vi "DrawText.vi"(0 "reference in":refnum<class "LcPictureBox.lvclass">, 1 "Origin":cluster{"X":sgl, "Y":sgl}, 2 "Alignment(Left,Top)":T2, 3 "Text":string, 5 "Error In":errorcluster, 6 "Font(Arial,14pts,Regular)":T1={"FontName"="Arial", "Size(Pts)"=14.0, "Style"=enum."Regular"}, 7 "Color(Black)":u32(colorbox), 8 "SmoothingMode((AntiAlias))":T3=enum."AntiAlias", 9 "Alpha(100%)":dbl=100.0 min=0.0 max=100.0 format="%#_g%%", 10 "BgColor(Transparent)":u32(colorbox)=16777216) -> (14 "reference out":refnum<class "LcPictureBox.lvclass">, 19 "Error Out":errorcluster)   [LabVIEW 2020, in "LcPictureBox.lvclass"]
uses:
  <userlib>/_LabVIEWCommon/LcPictureBox_class/LcPictureBox.lvclass
  <userlib>/_LabVIEWCommon/LcPictureBox_class/SmoothingMode.ctl
  <userlib>/_LabVIEWCommon/LcPictureBox_class/Font.ctl
  System.Drawing
  <userlib>/_LabVIEWCommon/LcPictureBox_class/LcPictureBox.lvclass/LcPictureBox.ctl
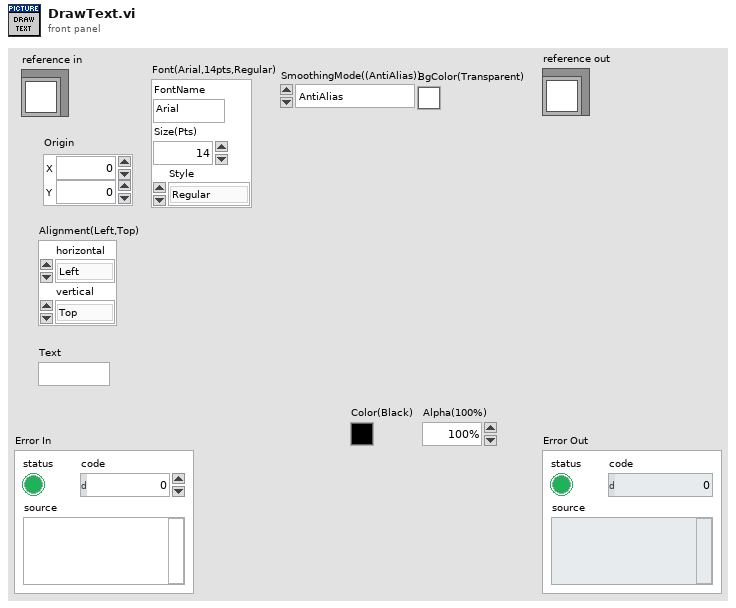
[diagram p1: front panel]
types:
  T1 = typedef "LcPictureBox.lvclass/Font.ctl" = cluster{"FontName":string, "Size(Pts)":dbl, "Style":enum16{"Regular", "Bold", "Italic", "Underline", "Strikeout"}}
  T2 = cluster{"horizontal":enum16{"Left", "Center", "Right"}, "vertical":enum16{"Top", "Center", "Bottom"}}
  T3 = typedef "LcPictureBox.lvclass/SmoothingMode.ctl" = enum16{"None", "HighSpeed", "HighQuality", "AntiAlias"}
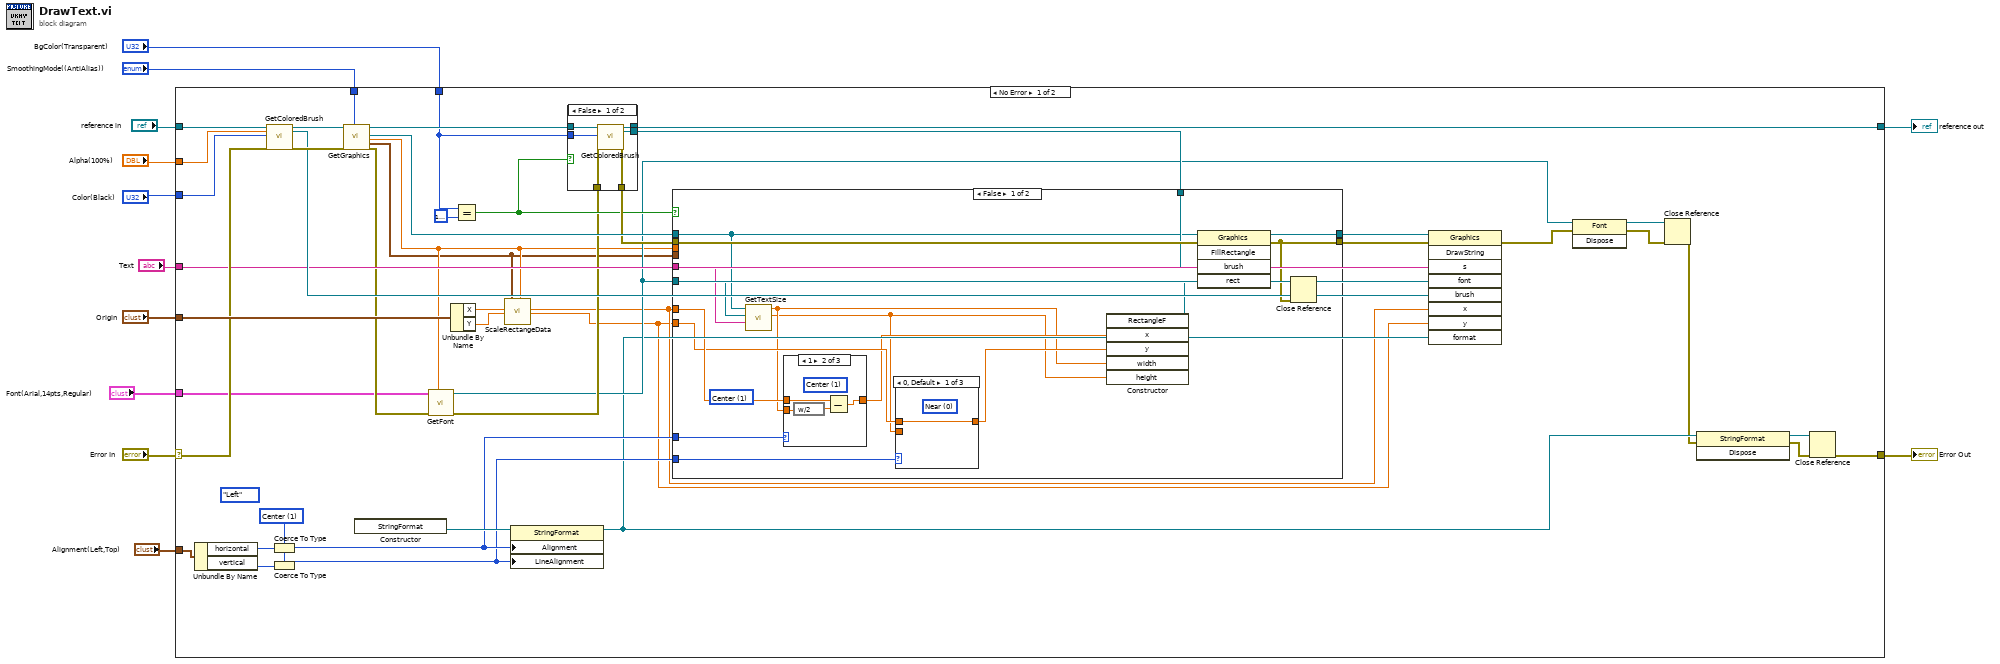
[diagram p0: block diagram]
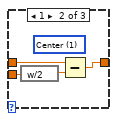
[diagram p2: hidden frame]
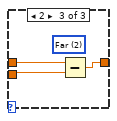
[diagram p3: hidden frame]
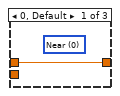
[diagram p4: hidden frame]
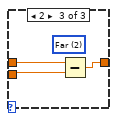
[diagram p5: hidden frame]
diagram:
  n1 = case shown="No Error" "Error In" {
    selector: "Error In" -> [w54 w101]
    tunnel: [w29 w101] -> w11
    tunnel: [w37 w100] -> w10
    tunnel: "reference in" -> [w56 w100]
    tunnel: "SmoothingMode((AntiAlias))" -> [w50 _]
    tunnel: "Color(Black)" -> [w52 _]
    tunnel: "Alpha(100%)" -> [w53 _]
    tunnel: "Origin" -> [w57 _]
    tunnel: "Text" -> [w48 _]
    tunnel: "Alignment(Left,Top)" -> [w45 _]
    tunnel: "Font(Arial,14pts,Regular)" -> [w41 _]
    tunnel: "BgColor(Transparent)" -> [w35 _]
    frame No Error {
      (unwired) enum16{"Left", "Center", "Right"}."Left" ("horizontal")
      w42 = 1 items=["Near", "Center", "Far"] ("Alignment")
      n2 = Unbundle By Name(w45) -> ("horizontal"=w44:enum16{"Left", "Center", "Right"}, "vertical"=w43:enum16{"Top", "Center", "Bottom"})
      n3 = call <userlib>:"GetColoredBrush.vi"("reference in"=w56, "Alpha(100%)"=w53, "Color(Black)"=w52, "Error In"=w54) -> ("reference out"=w55:refnum<class "LcPictureBox.lvclass">, "SolidBrushRef"=w49:refnum<k24>, "Error Out"=w51:errorcluster)  [unwired: 13 in]
      n4 = Coerce To Type(0:w44, 1:w42) -> (2:w31:i32)
      n5 = Coerce To Type(0:w43, 1:w42) -> (2:w30:i32)
      n6 = call <userlib>:"GetGraphics.vi"("LcPictureBox in"=w55, "error in (no error)"=w51, "SmoothingMode"=w50) -> ("LcPictureBox out"=w38:refnum<class "LcPictureBox.lvclass">, "Graphics"=w40:refnum<k24>, "Scale"=w16:dbl, "Offset"=w15:cluster{"x":sgl, "y":sgl}, "error out"=w47:errorcluster)  [unwired: 12 in]
      n7 = constructor class="StringFormat"() -> (reference out=w46:refnum<k24>)  [unwired: 3 in, 2 out]
      n8 = call <userlib>:"GetFont.vi"("Scale"=w16, "error in (no error)"=w47, "Font(Arial,14pts,Regular)"=w41) -> ("error out"=w32:errorcluster, "Font"=w28:refnum<k24>)  [unwired: 7 in]
      n9 = Unbundle By Name(w57) -> ("X"=w20:sgl, "Y"=w18:sgl)
      n10 = Equal?(x=w35, y=u32 16777216) -> (x = y?=w34:bool)
      n11 = call <userlib>:"ScaleRectangeData.vi"("X-In"=w20, "Y-In"=w18, "Offset(raw)"=w15, "Scale"=w16) -> ("X-Out"=w19:sgl, "Y-Out"=w17:sgl)  [unwired: 12 in, 2 out]
      n12 = property class="StringFormat"(reference=w46, "Alignment"=w31, "LineAlignment"=w30) -> (reference out=w24:refnum<k24>)  [unwired: 1 in, 1 out]
      n13 = case shown="False" w34 {
        tunnel: w38 -> [w97 w99]
        tunnel: [w96 w99] -> w37
        tunnel: w32 -> [w95 w98]
        tunnel: [w94 w98] -> w36
        tunnel: w35 -> [w93 _]
        tunnel: [w92 _] -> w33
        frame False {
          n14 = call <userlib>:"GetColoredBrush.vi"("reference in"=w97, "Color(Black)"=w93, "Error In"=w95) -> ("reference out"=w96:refnum<class "LcPictureBox.lvclass">, "SolidBrushRef"=w92:refnum<k24>, "Error Out"=w94:errorcluster)  [unwired: 14 in]
        }
        frame True {
        }
      }
      n15 = case shown="False" w34 {
        tunnel: w36 -> [w73 w90]
        tunnel: w40 -> [w68 w91]
        tunnel: [w72 w91] -> w14
        tunnel: [w63 w90] -> w13
        tunnel: w33 -> [w71 _]
        tunnel: w48 -> [w69 _]
        tunnel: w28 -> [w70 _]
        tunnel: w19 -> [w66 _]
        tunnel: w17 -> [w64 _]
        tunnel: w31 -> [w67 _]
        tunnel: w30 -> [w65 _]
        tunnel: w15 -> [_ _]
        tunnel: w16 -> [_ _]
        frame False {
          (unwired) 1 items=["Near", "Center", "Far"] ("Alignment")
          n16 = call <userlib>:"GetTextSize.vi"("Text"=w69, "Font"=w70, "Graphics"=w68) -> ("Height"=w58:sgl, "Width"=w59:sgl)  [unwired: 6 in, 1 out]
          n17 = case shown="1" w67 {
            tunnel: w59 -> [_ w86 w87]
            tunnel: w66 -> [w82 w85 w89]
            tunnel: [w82 w83 w88] -> w61
            frame 0, Default {
              (unwired) 0 items=["Near", "Center", "Far"] ("Alignment")
            }
            frame 1 {
              (unwired) 1 items=["Near", "Center", "Far"] ("Alignment")
              n18 = expression code="w/2"(w86) -> (w84:sgl)
              n19 = Subtract(x=w85, y=w84) -> (x-y=w83:sgl)
            }
            frame 2 {
              (unwired) 2 items=["Near", "Center", "Far"] ("Alignment")
              n20 = Subtract(x=w89, y=w87) -> (x-y=w88:sgl)
            }
          }
          n21 = case shown="0, Default" w65 {
            tunnel: w58 -> [_ w78 w79]
            tunnel: w64 -> [w74 w77 w81]
            tunnel: [w74 w75 w80] -> w60
            frame 0, Default {
              (unwired) 0 items=["Near", "Center", "Far"] ("Alignment")
            }
            frame 1 {
              (unwired) 1 items=["Near", "Center", "Far"] ("Alignment")
              n22 = expression code="w/2"(w78) -> (w76:sgl)
              n23 = Subtract(x=w77, y=w76) -> (x-y=w75:sgl)
            }
            frame 2 {
              (unwired) 2 items=["Near", "Center", "Far"] ("Alignment")
              n24 = Subtract(x=w81, y=w79) -> (x-y=w80:sgl)
            }
          }
          n25 = constructor class="RectangleF"("x"=w61, "y"=w60, "width"=w59, "height"=w58) -> (reference out=w62:refnum<k24>)  [unwired: 3 in, 6 out]
          n26 = invoke class="Graphics" method="FillRectangle"(reference=w68, error in=w73, "brush"=w71, "rect"=w62) -> (reference out=w72:refnum<k24>, error out=w63:errorcluster)  [unwired: 1 in, 3 out]
          n27 = Close Reference(reference=w62, error in (no error)=w63) -> ()  [unwired: 1 out]
        }
        frame True {
        }
      }
      n28 = invoke class="Graphics" method="DrawString"(reference=w14, error in=w13, "s"=w48, "font"=w28, "brush"=w49, "x"=w19, "y"=w17, "format"=w24) -> (error out=w26:errorcluster)  [unwired: 1 in, 8 out]
      n29 = invoke class="Font" method="Dispose"(reference=w28, error in=w26) -> (reference out=w27:refnum<k24>, error out=w25:errorcluster)  [unwired: 1 in, 1 out]
      n30 = Close Reference(reference=w27, error in (no error)=w25) -> (error out=w22:errorcluster)
      n31 = invoke class="StringFormat" method="Dispose"(reference=w24, error in=w22) -> (reference out=w23:refnum<k24>, error out=w21:errorcluster)  [unwired: 1 in, 1 out]
      n32 = Close Reference(reference=w23, error in (no error)=w21) -> (error out=w29:errorcluster)
    }
    frame Error {
    }
  }
  "Error Out" <- w11
  "reference out" <- w10
